vi "Remove_common_prefix.vi"(2 "Max String Length":i32=32, 3 "Array in":string[](array[string])) -> (1 "Array out":string[](array[string]))   [LabVIEW 2014]
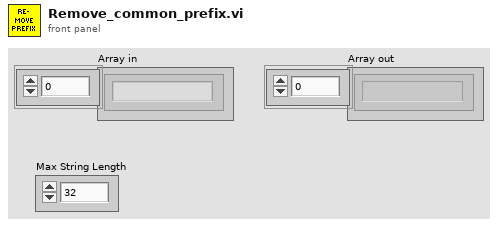
[diagram p1: front panel]
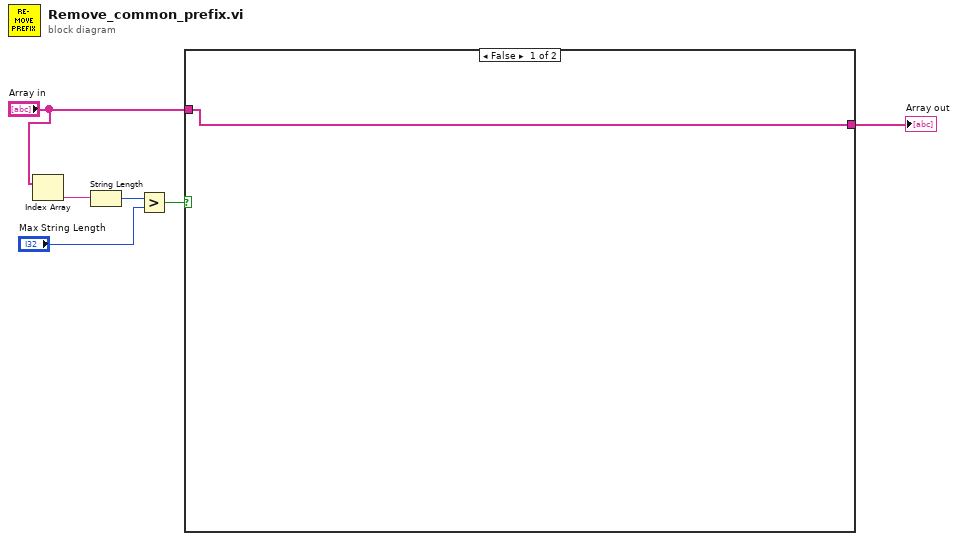
[diagram p0: block diagram]
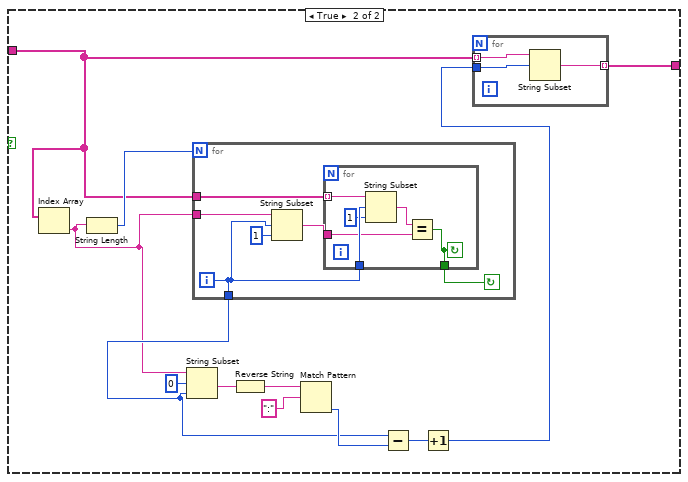
[diagram p2: hidden frame]
diagram:
  n1 = Index Array(array="Array in") -> (element=w5:string)  [unwired: 1 in]
  n2 = String Length(string=w5) -> (length=w3:i32)
  n3 = Greater?(x=w3, y="Max String Length") -> (0:w2:bool)
  n4 = case shown="False" w2 {
    tunnel: [w7 w17] -> w6
    tunnel: "Array in" -> [w7 w8]
    frame False {
    }
    frame True {
      n5 = Index Array(array=w8) -> (element=w11:string)  [unwired: 1 in]
      n6 = String Length(string=w11) -> (length=w9:i32)
      n7 = for {
        N: w9 -> [_]
        tunnel: w8 -> [w28]
        tunnel: w11 -> [w26]
        tunnel: [w23] -> w15
        i -> [w23]
        stop <- w24 continue-if-true
        n8 = String Subset(string=w26, offset (0)=w23, length (rest)=1 ("length (rest)")) -> (substring=w25:string)
        n9 = for {
          tunnel: w23 -> [w34]
          tunnel: w28 -> [w32] mode=indexing
          tunnel: w25 -> [w30]
          tunnel: [w29] -> w24
          stop <- w29 continue-if-true
          n10 = String Subset(string=w32, offset (0)=w34, length (rest)=1 ("length (rest)")) -> (substring=w31:string)
          n11 = Equal?(x=w31, y=w30) -> (x = y?=w29:bool)
        }
      }
      n12 = String Subset(string=w11, offset (0)=0, length (rest)=w15) -> (substring=w12:string)
      n13 = Reverse String(1:w12) -> (0:w13:string)
      n14 = Match Pattern(string=w13, regular expression=":") -> (offset past match=w16:i32)  [unwired: 1 in, 3 out]
      n15 = Subtract(x=w15, y=w16) -> (x-y=w18:i32)
      n16 = Increment(x=w18) -> (x+1=w19:i32)
      n17 = for {
        tunnel: w19 -> [w22]
        tunnel: w8 -> [w21] mode=indexing
        tunnel: [w20] -> w17 mode=indexing
        n18 = String Subset(string=w21, offset (0)=w22) -> (substring=w20:string)  [unwired: 1 in]
      }
    }
  }
  "Array out" <- w6
